vi "Folder.vi"(11 "Folders":T1) -> (2 "found?":bool, 3 "FolderPath":path)   [LabVIEW 2015]
uses:
  <vilib>/Utility/config.llb/NI_LVConfig.lvlib
  <vilib>/Utility/config.llb/Read Key (Boolean).vi
  Folders.ctl
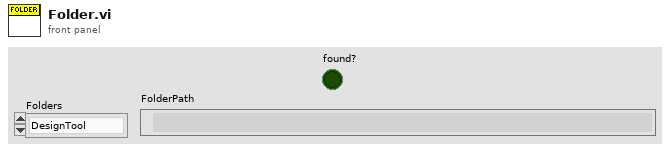
[diagram p1: front panel]
types:
  T1 = typedef "Folders.ctl" = enum16{"DesignTool", "RequestedDesigns", "CompletedDesigns"}
  T2 = typedef "NI_LVConfig.lvlib/Config Data RefNum.ctl" = refnum<k1>
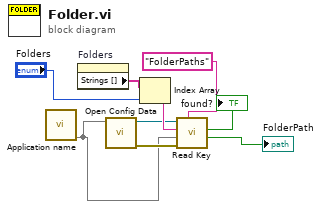
[diagram p0: block diagram]
diagram:
  n1 = call "Application name.vi"() -> (0:w4)  [unwired: 4 in, 3 out]
  n2 = property on="Folders" class="Enum (strict)"() -> ("Strings []"=w8:string[])  [unwired: 2 in, 2 out]
  n3 = call <vilib>:"Open Config Data.vi"("configuration file path"=w4) -> ("error out"=w9:errorcluster, "refnum"=w3:T2)  [unwired: 8 in, 1 out]
  n4 = Index Array(array=w8, index="Folders") -> (element=w6:string)
  n5 = call-poly <vilib>:"Read Key.vi"("section"="FolderPaths", "error in (no error)"=w9, "default value"=w4, "key"=w6, "refnum"=w3) -> ("value"=→"FolderPath":bool, "found?"=→"found?":bool)  [unwired: 3 in, 2 out]
